vi "fm.vi"() -> ()   [LabVIEW 2018]
uses:
  <vilib>/measure/NI_MABase.lvlib
panel:
  out "Waveform Chart":waveform(dbl)(graph)
  out "Carrier wave":waveform(dbl)(graph)
  out "FM modulated":dynamicdata(graph)
  in  "Fc":dbl(slide) scale=0.0..1000000.0
  in  "Deviation":dbl(slide) scale=0.0..10.0
  in  "Fm":dbl(slide) scale=0.0..100000.0
  in  "stop":bool
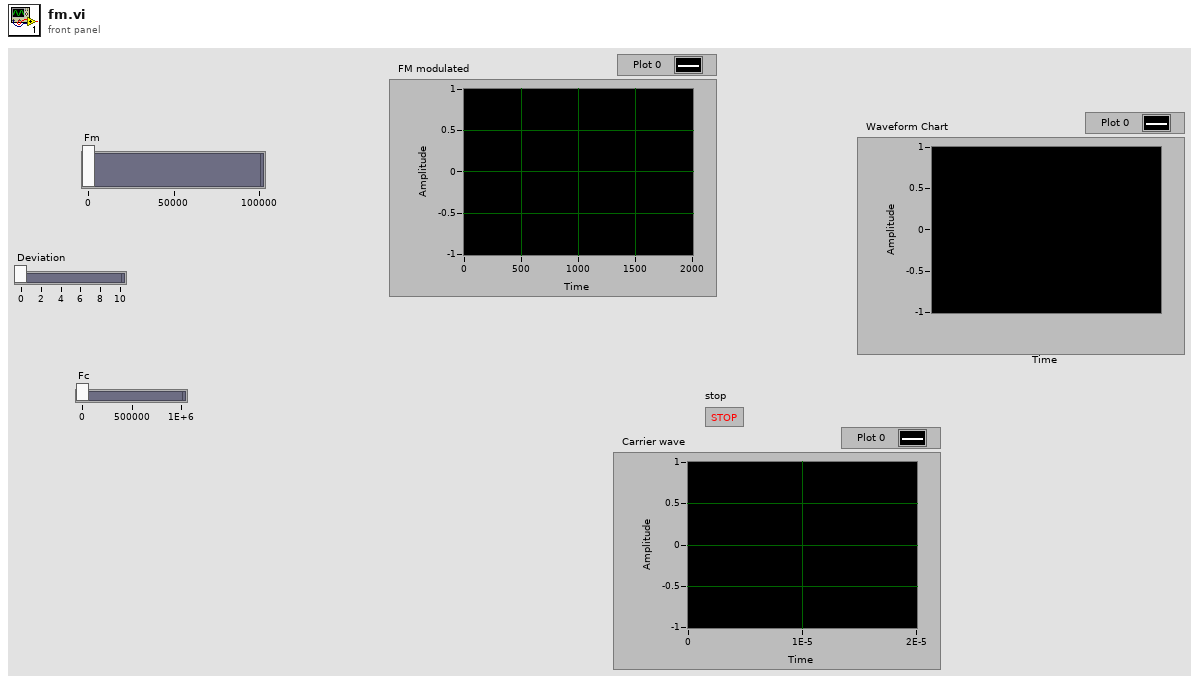
[diagram p1: front panel]
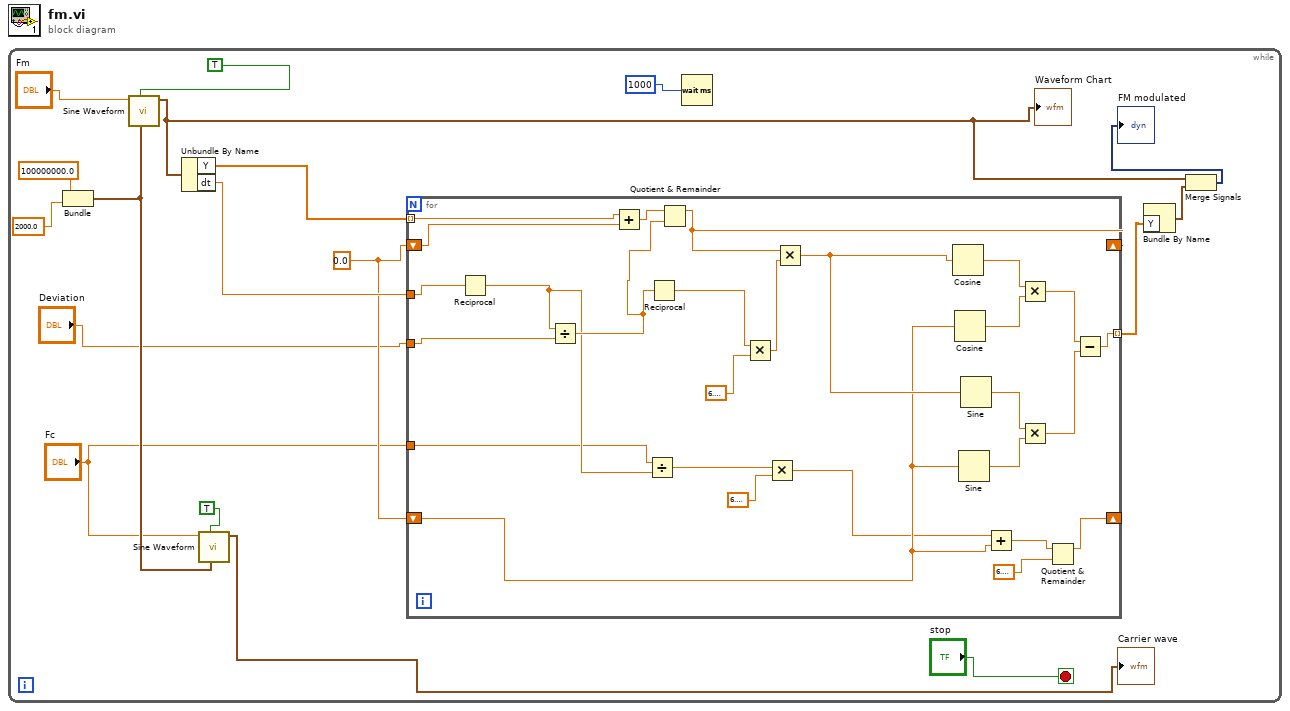
[diagram p0: block diagram]
diagram:
  n1 = while {
    stop <- "stop" stop-if-true
    w8 = 0.0
    n2 = Bundle(100000000.0, 2000.0) -> (w12:cluster{dbl, dbl})  [unwired: 1 in]
    n3 = call <vilib>:"Sine Waveform.vi"("sampling info"=w12, "reset signal"=TRUE, "frequency"="Fm") -> ("signal out"=w2:waveform(dbl))  [unwired: 7 in, 1 out]
    "Waveform Chart" <- w2
    n4 = Unbundle By Name(w2) -> ("Y"=w10:dbl[], "dt"=w9:dbl)
    n5 = call <vilib>:"Sine Waveform.vi"("sampling info"=w12, "reset signal"=TRUE, "frequency"="Fc") -> ("signal out"=→"Carrier wave":waveform(dbl))  [unwired: 7 in, 1 out]
    n6 = for {
      shift-right: [w33] -> _
      shift-left: w8 -> [w44]
      shift-right: [w22] -> _
      shift-left: w8 -> [w26]
      tunnel: w10 -> [w45] mode=indexing
      tunnel: w9 -> [w43]
      tunnel: "Deviation" -> [w40]
      tunnel: "Fc" -> [w27]
      tunnel: [w19] -> w5 mode=indexing
      n7 = Reciprocal(x=w43) -> (1/x=w39:dbl)
      n8 = Divide(x=w39, y=w40) -> (x/y=w41:dbl)
      n9 = Add(x=w45, y=w44) -> (x+y=w42:dbl)
      n10 = Divide(x=w27, y=w39) -> (x/y=w38:dbl)
      n11 = Reciprocal(x=w41) -> (1/x=w35:dbl)
      n12 = Quotient & Remainder(x=w42, y=w41) -> (x-y*floor(x/y)=w33:dbl)  [unwired: 1 out]
      n13 = Multiply(x=w35, y=6.283185307179586) -> (x*y=w34:dbl)
      n14 = Multiply(x=w38, y=6.283185307179586) -> (x*y=w25:dbl)
      n15 = Multiply(x=w33, y=w34) -> (x*y=w30:dbl)
      n16 = Cosine(x=w30) -> (cos(x)=w31:dbl)
      n17 = Cosine(x=w26) -> (cos(x)=w32:dbl)
      n18 = Sine(x=w26) -> (sin(x)=w29:dbl)
      n19 = Sine(x=w30) -> (sin(x)=w28:dbl)
      n20 = Add(x=w25, y=w26) -> (x+y=w24:dbl)
      n21 = Multiply(x=w31, y=w32) -> (x*y=w21:dbl)
      n22 = Multiply(x=w28, y=w29) -> (x*y=w20:dbl)
      n23 = Quotient & Remainder(x=w24, y=6.283185307179586) -> (x-y*floor(x/y)=w22:dbl)  [unwired: 1 out]
      n24 = Subtract(x=w21, y=w20) -> (x-y=w19:dbl)
    }
    n25 = Wait (ms)(milliseconds to wait=u32 1000 ("millisecond timer value")) -> ()  [unwired: 1 out]
    n26 = Bundle By Name("Y"=w5) -> (w3:waveform(dbl))  [unwired: 1 in]
    n27 = Merge Signals(w2, w3) -> (→"FM modulated":dynamicdata)
  }
